vi "DesignPatterns_GetAttributesAndMethods.vi"(11 "ClassText":string) -> (1 "Methods":T2[](array[typedef]), 2 "Attributes":T1[](array[typedef]), 3 "Desciption":string)   [LabVIEW 2014]
uses:
  <resource>/Framework/Providers/Open_GDS/UML/DesignPattern/SubVIs/DesignPatterns_Method.ctl
  <resource>/Framework/Providers/Open_GDS/UML/DesignPattern/SubVIs/DesignPatterns_Attribute.ctl
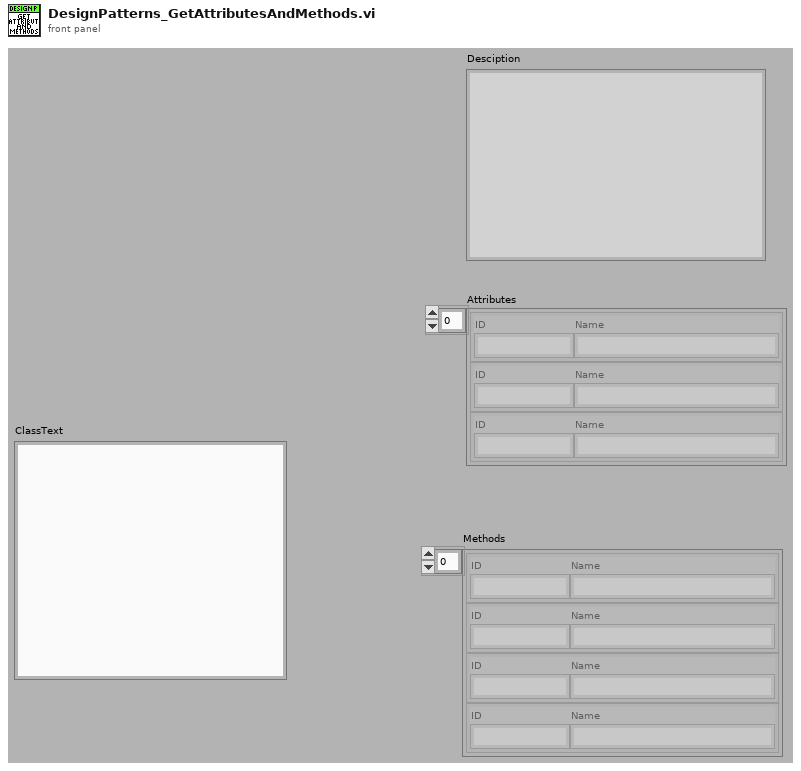
[diagram p1: front panel]
types:
  T1 = typedef "DesignPatterns_Attribute.ctl" = cluster{"ID":string, "Name":string}
  T2 = typedef "DesignPatterns_Method.ctl" = cluster{"ID":string, "Name":string}
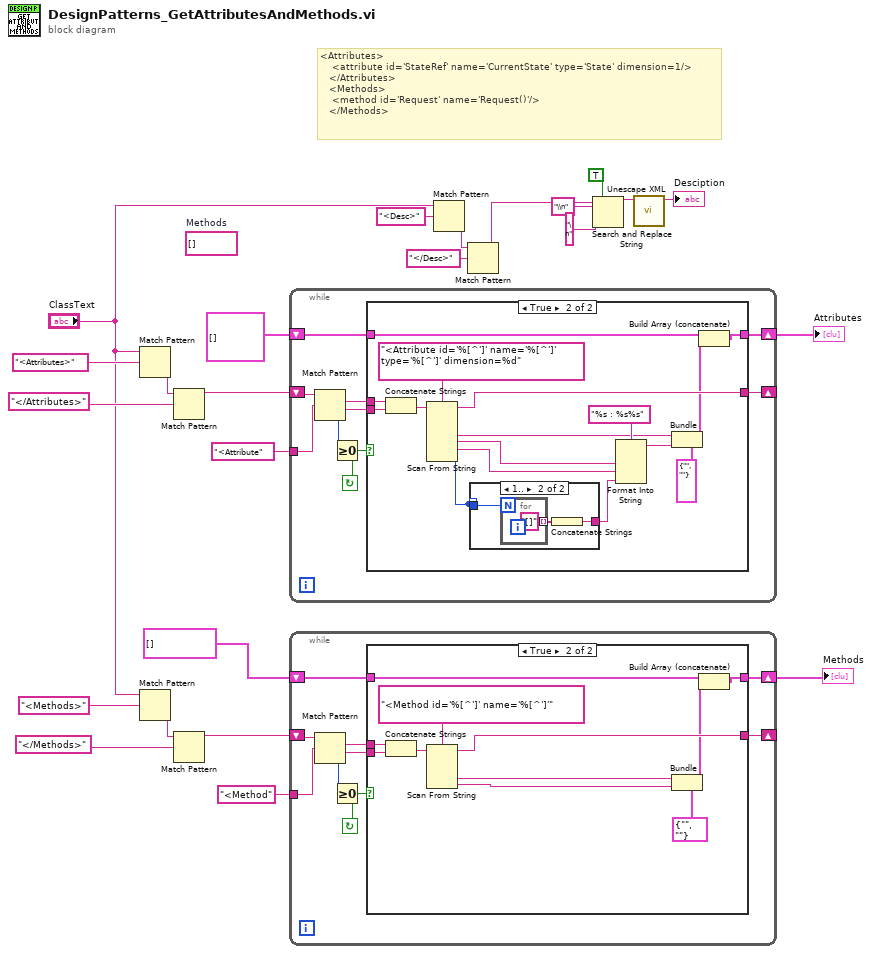
[diagram p0: block diagram]
diagram:
  (unwired) string[] []  # Methods
  # "<Attributes>\n\t\t\t\t<attribute id='StateRef' name='CurrentState' type='State' dimension=1/>\n\t\t\t</Attributes>\n\t\t\t<Methods>\n\t\t\t\t<method id='Request' name='Request()'/>\n\t\t\t</Methods>"
  n1 = Match Pattern(string="ClassText", regular expression="<Attributes>") -> (after substring=w23:string)  [unwired: 4 out]
  n2 = Match Pattern(string="ClassText", regular expression="<Methods>") -> (after substring=w15:string)  [unwired: 4 out]
  n3 = Match Pattern(string=w23, regular expression="</Attributes>") -> (before substring=w21:string)  [unwired: 4 out]
  n4 = Match Pattern(string=w15, regular expression="</Methods>") -> (before substring=w16:string)  [unwired: 4 out]
  n5 = while {
    shift-right: [w27] -> _
    shift-left: w21 -> [w31]
    tunnel: "<Attribute" ("regular expression") -> [w30]
    shift-right: [w25] -> w19
    shift-left: T1[] [] ("Attributes") -> [w26]
    stop <- w28 continue-if-true
    n6 = Match Pattern(string=w31, regular expression=w30) -> (match substring=w32:string, after substring=w33:string, offset past match=w29:i32)  [unwired: 2 out]
    n7 = Greater Or Equal To 0?(x=w29) -> (x >= 0?=w28:bool)
    n8 = case shown="True" w28 {
      tunnel: w33 -> [_ w49]
      tunnel: w32 -> [_ w48]
      tunnel: [_ w47] -> w27
      tunnel: w26 -> [w34 w45]
      tunnel: [w34 w44] -> w25
      frame False {
      }
      frame True {
        n9 = Concatenate Strings(w48, w49) -> (w50:string)
        n10 = Scan From String(format string="<Attribute id='%[^']' name='%[^']' type='%[^']' dimension=%d", input string=w50) -> (remaining string=w47:string, output 1=w38:string, output 2=w43:string, output 3=w41:string, output 4=w35:i32)  [unwired: 2 in, 6 out]
        n11 = case shown="1.." w35 {
          tunnel: [_ w52] -> w40
          tunnel: w35 -> [_ w51]
          frame Default {
          }
          frame 1.. {
            n12 = for {
              N: w51 -> [_]
              tunnel: ["[]" ("format string")] -> w53 mode=indexing
            }
            n13 = Concatenate Strings(w53) -> (w52:string)
          }
        }
        n14 = Format Into String(format string="%s : %s%s", w43, w41, w40) -> (resulting string=w39:string)  [unwired: 2 in, 1 out]
        n15 = Bundle(cluster=T1 {"ID"="", "Name"=""}, "ID"=w38, "Name"=w39) -> (w37:T1)
        n16 = Build Array (concatenate)(w45, w37) -> (w44:T1[])
      }
    }
  }
  "Attributes" <- w19
  n17 = while {
    shift-right: [w57] -> _
    shift-left: w16 -> [w61]
    tunnel: "<Method" ("regular expression") -> [w60]
    shift-right: [w55] -> w12
    shift-left: T2[] [] ("Methods") -> [w56]
    stop <- w58 continue-if-true
    n18 = Match Pattern(string=w61, regular expression=w60) -> (match substring=w62:string, after substring=w63:string, offset past match=w59:i32)  [unwired: 2 out]
    n19 = Greater Or Equal To 0?(x=w59) -> (x >= 0?=w58:bool)
    n20 = case shown="True" w58 {
      tunnel: w63 -> [_ w74]
      tunnel: w62 -> [_ w73]
      tunnel: [_ w72] -> w57
      tunnel: w56 -> [w64 w70]
      tunnel: [w64 w69] -> w55
      frame False {
      }
      frame True {
        n21 = Concatenate Strings(w73, w74) -> (w75:string)
        n22 = Scan From String(format string="<Method id='%[^']' name='%[^']'", input string=w75) -> (remaining string=w72:string, output 1=w68:string, output 2=w65:string)  [unwired: 2 in, 4 out]
        n23 = Bundle(cluster=T2 {"ID"="", "Name"=""}, "ID"=w68, "Name"=w65) -> (w67:T2)
        n24 = Build Array (concatenate)(w70, w67) -> (w69:T2[])
      }
    }
  }
  "Methods" <- w12
  n25 = Match Pattern(string="ClassText", regular expression="<Desc>") -> (after substring=w10:string)  [unwired: 4 out]
  n26 = Match Pattern(string=w10, regular expression="</Desc>") -> (before substring=w3:string)  [unwired: 4 out]
  n27 = Search and Replace String(replace all?=TRUE ("replace all? (F)"), input string=w3, search string="\\n", replace string="\n" ("replace string (\"\")")) -> (result string=w4:string)  [unwired: 1 in, 6 out]
  n28 = call <vilib>:"Unescape XML.vi"("XML String In"=w4) -> ("XML String Out"=→"Desciption":string)  [unwired: 1 in, 9 out]
